vi "SENS_CORR_EXT_AUTO_MEAS.vi"(0 "VISA IN":refnum<visa-resource-name>, 1 "Standard":string, 5 "error in":errorcluster, 7 "Channel":i32) -> (14 "VISA Out":refnum<visa-resource-name>, 19 "error out":errorcluster)   [LabVIEW 2018, in "PNA-X.lvlib"]
doc: "SENSe<cnum>:CORRection:EXTension:AUTO:MEASure <char> \n1701\n\n(Write-only) Measures either an OPEN or SHORT standard. When this command is sent, the PNA \nacquires the measurement with which to set automatic port extensions. Learn more about which \nstandard to measure. \nParameters \n<cnum> Any existing channel number. If unspecified, value is set to 1 \n<char> Standard to be measured. Choose from: \nOPEN Measure OPEN standard \nSHORt Measure SHORT standard \nExamples SENS:CORR:EXT:AUTO:MEAS OPEN \nsense2:correction:extension:auto:measure short \nQuery Syntax Not Applicable \nDefault Not Applicable"
uses:
  PNA-X.lvlib
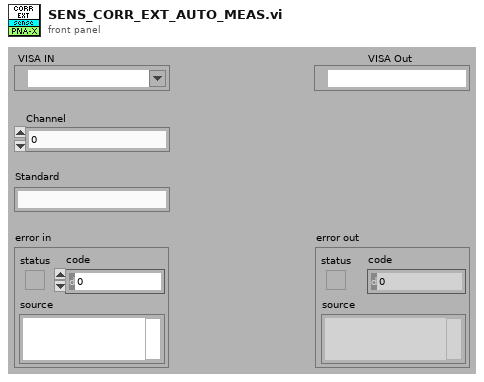
[diagram p1: front panel]
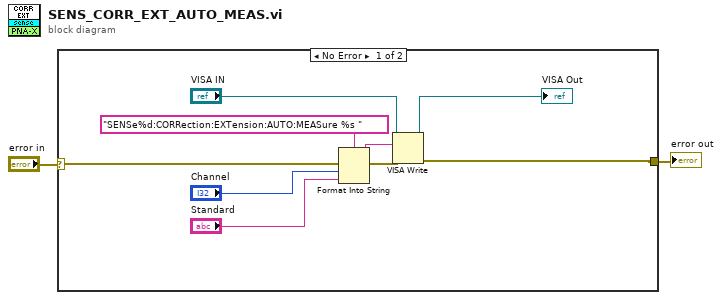
[diagram p0: block diagram]
diagram:
  n1 = case shown="No Error" "error in" {
    selector: "error in" -> [w11 w12]
    tunnel: [w6 w12] -> w1
    frame No Error {
      n2 = Format Into String(format string="SENSe%d:CORRection:EXTension:AUTO:MEASure %s " ("Cmdline"), error in=w11, "Channel", "Standard") -> (resulting string=w9:string, error out=w10:errorcluster)  [unwired: 1 in]
      n3 = VISA Write(VISA resource name="VISA IN", write buffer=w9, error in (no error)=w10) -> (VISA resource name out=→"VISA Out":refnum<visa-resource-name>, error out=w6:errorcluster)  [unwired: 1 out]
    }
    frame Error {
    }
  }
  "error out" <- w1
